vi "computeDeconMatrix.vi"(8 "error in (no error)":errorcluster, 11 "LaguerreDeconClass in":refnum<class "LaguerreDeconEngineClass.lvclass">) -> (0 "error out":errorcluster, 3 "LaguerreDeconClass out":refnum<class "LaguerreDeconEngineClass.lvclass">)   [LabVIEW 2024, in "LaguerreDeconEngineClass.lvclass"]
uses:
  LaguerreDeconEngineClass.lvclass
  LaguerreDeconEngineClass.lvclass/LaguerreDeconEngineClass.ctl
  LaguerreDeconLib.lvlib
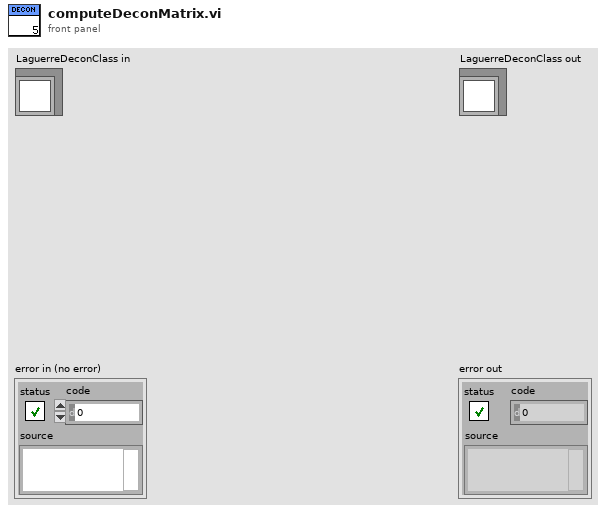
[diagram p1: front panel]
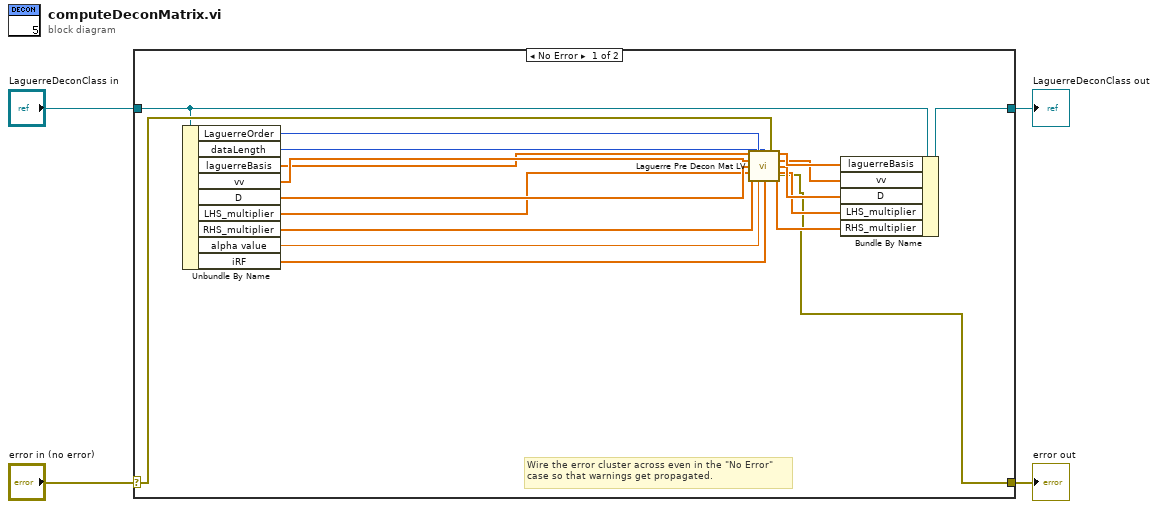
[diagram p0: block diagram]
diagram:
  n1 = case shown="No Error" "error in (no error)" {
    selector: "error in (no error)" -> [w16 w24]
    tunnel: [w15 w24] -> w3
    tunnel: [w22 w23] -> w1
    tunnel: "LaguerreDeconClass in" -> [w14 w23]
    frame No Error {
      # "Wire the error cluster across even in the \"No Error\"\ncase so that warnings get propagated."
      n2 = Unbundle By Name(w14) -> ("LaguerreOrder"=w8:u32, "dataLength"=w7:u32, "laguerreBasis"=w12:dbl[], "vv"=w13:dbl[], "D"=w11:dbl[], "LHS_multiplier"=w10:dbl[], "RHS_multiplier"=w9:dbl[], "alpha value"=w6:dbl, "iRF"=w5:dbl[])
      n3 = call "Laguerre Pre Decon Mat LV.vi"("laguerreBasis_array in"=w12, "laguerreOrder"=w8, "dataLength"=w7, "error in (no error)"=w16, "vv_array in"=w13, "D_mat_array in"=w11, "LHS_multiplier_array in"=w10, "RHS_multiplier_array in"=w9, "alpha"=w6, "iRF_array"=w5) -> ("laguerreBasis_array out"=w21:dbl[], "vv_array out"=w20:dbl[], "D_mat_array out"=w19:dbl[], "LHS_multiplier_array out"=w18:dbl[], "error out"=w15:errorcluster, "RHS_multiplier_array out"=w17:dbl[])
      n4 = Bundle By Name(cluster=w14, "laguerreBasis"=w21, "vv"=w20, "D"=w19, "LHS_multiplier"=w18, "RHS_multiplier"=w17) -> (w22:refnum<class "LaguerreDeconEngineClass.lvclass">)
    }
    frame Error {
    }
  }
  "error out" <- w3
  "LaguerreDeconClass out" <- w1
